vi "FromRepo.vi"(8 "error in":errorcluster, 9 "from repo cluster":T2, 10 "repository in":refnum<class "NISE_CEF_Repository.lvclass">, 11 "node in":refnum<class "NISE_CEF_Node.lvclass">) -> (0 "error out":errorcluster, 2 "repository out":refnum<class "NISE_CEF_Repository.lvclass">, 3 "node":T1)   [LabVIEW 2013, in "NISE_CEF_Node.lvclass"]
doc: "Grabs information from the Repo and stores it in the nodes."
uses:
  NISE_CEF_Node.lvclass
  Repository/NISE_CEF_Repository.lvclass
  FromRepoCluster.ctl
  NodeRef.ctl
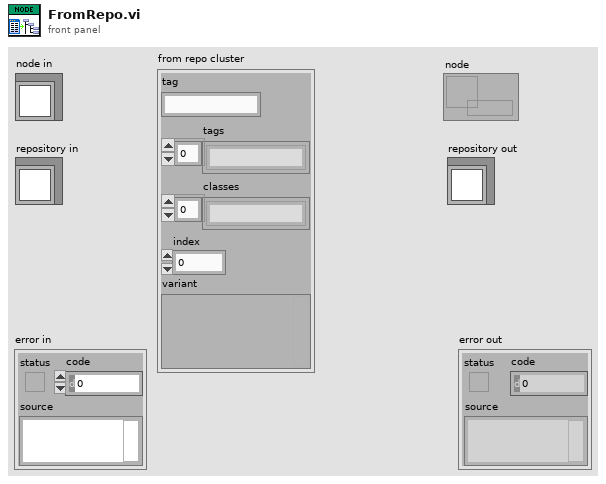
[diagram p1: front panel]
types:
  T1 = typedef "NISE_CEF_Node.lvclass/NodeRef.ctl" = refnum<data-value>
  T2 = typedef "NISE_CEF_Node.lvclass/FromRepoCluster.ctl" = cluster{"tag":string, "tags":string[], "classes":string[], "index":i32, "variant":variant}
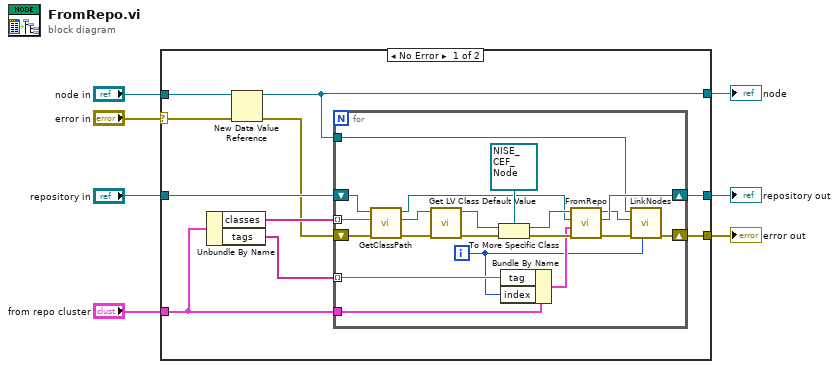
[diagram p0: block diagram]
diagram:
  n1 = case shown="No Error" "error in" {
    selector: "error in" -> [w9 w39]
    tunnel: [w16 w39] -> w6
    tunnel: "node in" -> [w14 _]
    tunnel: "repository in" -> [w10 w38]
    tunnel: [w15 w38] -> w3
    tunnel: "from repo cluster" -> [w11 _]
    tunnel: [w13 _] -> w1
    frame No Error {
      n2 = Unbundle By Name(w11) -> ("classes"=w17:string[], "tags"=w12:string[])
      n3 = New Data Value Reference(data value=w14, error in=w9) -> (data value reference=w13:refnum<data-value>, error out=w8:errorcluster)
      n4 = for {
        tunnel: w17 -> [w18] mode=indexing
        shift-right: [w32] -> w15
        shift-left: w10 -> [w23]
        shift-right: [w28] -> w16
        shift-left: w8 -> [w22]
        tunnel: w13 -> [w30]
        tunnel: w12 -> [w26] mode=indexing
        tunnel: w11 -> [w25]
        i -> [w24]
        n5 = call-dynamic "GetClassPath.vi"("error in"=w22, "class name"=w18, "Repository in"=w23) -> ("error out"=w21:errorcluster, "class path"=w20:path, "Repository out"=w19:refnum<class "NISE_CEF_Repository.lvclass">)  [unwired: 6 in]
        n6 = call <vilib>:"Get LV Class Default Value.vi"("error in (no error)"=w21, "class path"=w20) -> ("error out"=w35:errorcluster, "object"=w36:refnum<class>)  [unwired: 8 in]
        n7 = To More Specific Class(target class=refnum<class "NISE_CEF_Node.lvclass"> refnum ("node.lvclass"), reference=w36, error in=w35) -> (specific class reference=w34:refnum<class "NISE_CEF_Node.lvclass">, error out=w33:errorcluster)
        n8 = Bundle By Name(cluster=w25, "tag"=w26, "index"=w24) -> (w27:T2)
        n9 = call-dynamic "FromRepo.vi"("error in"=w33, "from repo cluster"=w27, "repository in"=w19, "node in"=w34) -> ("error out"=w29:errorcluster, "repository out"=w32:refnum<class "NISE_CEF_Repository.lvclass">, "node"=w31:T1)  [unwired: 5 in]
        n10 = call "LinkNodes.vi"("index"=w24, "error in"=w29, "child in"=w31, "parent in"=w30) -> ("error out"=w28:errorcluster)  [unwired: 5 in, 2 out]
      }
    }
    frame Error {
    }
  }
  "error out" <- w6
  "repository out" <- w3
  "node" <- w1
